vi "ElevatedPass.vi"(7 "PassState":T1, 8 "error in (no error)":errorcluster) -> (0 "error out":errorcluster)   [LabVIEW 2013]
doc: "Automatically performs the \"Elevated Pass\" maneuver."
uses:
  PassState.ctl
  RollerAction.ctl
  DoubleSolenoidAction.ctl
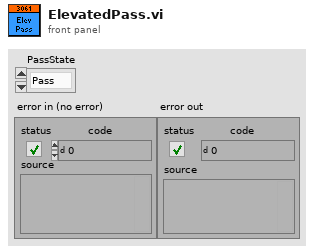
[diagram p1: front panel]
types:
  T1 = typedef "PassState.ctl" = enum16{"Pass", "Stop"}
  T2 = typedef "DoubleSolenoidAction.ctl" = enum16{"Init", "Middle", "In", "Out"}
  T3 = typedef "RollerAction.ctl" = enum16{"Init", "Off", "Forward", "Reverse"}
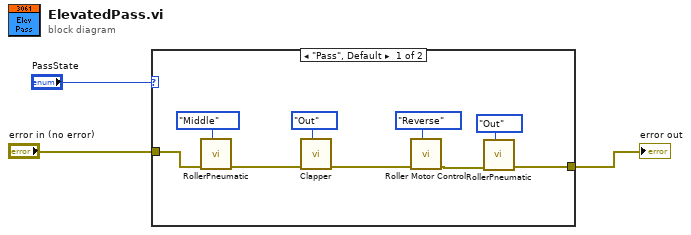
[diagram p0: block diagram]
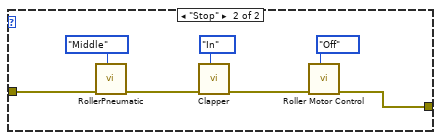
[diagram p2: hidden frame]
diagram:
  n1 = case shown="\"Pass\", Default" "PassState" {
    tunnel: "error in (no error)" -> [w6 w14]
    tunnel: [w5 w13] -> w2
    frame "Pass", Default {
      n2 = call "RollerPneumatic.vi"("State"=DoubleSolenoidAction."Middle", "Error in"=w6) -> ("Error out"=w8:errorcluster)  [unwired: 9 in]
      n3 = call "Clapper.vi"("State"=DoubleSolenoidAction."Out", "Error in"=w8) -> ("Error out"=w10:errorcluster)  [unwired: 9 in]
      n4 = call "Roller Motor Control.vi"("Action"=RollerAction."Reverse", "Error in"=w10) -> ("Error out"=w7:errorcluster)  [unwired: 9 in]
      n5 = call "RollerPneumatic.vi"("State"=DoubleSolenoidAction."Out", "Error in"=w7) -> ("Error out"=w5:errorcluster)  [unwired: 9 in]
    }
    frame "Stop" {
      n6 = call "RollerPneumatic.vi"("State"=DoubleSolenoidAction."Middle", "Error in"=w14) -> ("Error out"=w15:errorcluster)  [unwired: 9 in]
      n7 = call "Clapper.vi"("State"=DoubleSolenoidAction."In", "Error in"=w15) -> ("Error out"=w16:errorcluster)  [unwired: 9 in]
      n8 = call "Roller Motor Control.vi"("Action"=RollerAction."Off", "Error in"=w16) -> ("Error out"=w13:errorcluster)  [unwired: 9 in]
    }
  }
  "error out" <- w2
